vi "WriteConnInfoUSB.vi"(8 "error in (no error)":errorcluster, 9 "hostname":string="ConnectionInfo.json", 10 "path":path, 11 "connection info":T1) -> (0 "error out":errorcluster)   [LabVIEW 2017, in "USBDrive.lvlib"]
uses:
  <vilib>/addons/InsightCM/Devices/Shared/Common/USBDrive/USBDrive.lvlib
  <vilib>/addons/InsightCM/MessageBus/Base/controls/ConnectionInfo.ctl
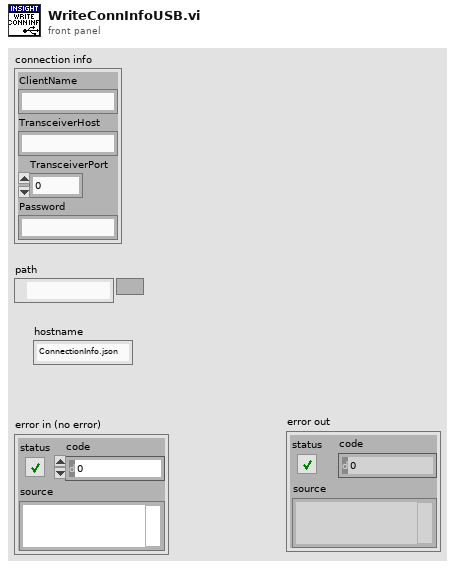
[diagram p1: front panel]
types:
  T1 = typedef "ConnectionInfo.ctl" = cluster{"ClientName":string, "TransceiverHost":string, "TransceiverPort":u16, "Password":string}
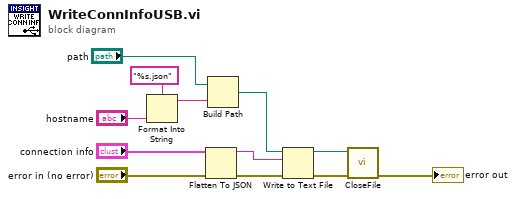
[diagram p0: block diagram]
diagram:
  n1 = Format Into String(format string="%s.json", "hostname") -> (resulting string=w8:string)  [unwired: 2 in, 1 out]
  n2 = Flatten To JSON(anything="connection info", error in (no error)="error in (no error)") -> (JSON string=w9:string, 11:w12:errorcluster)  [unwired: 1 in]
  n3 = Build Path(base path="path", name or relative path=w8) -> (appended path=w10:path)
  n4 = Write to Text File(file (use dialog)=w10, text=w9, error in=w12) -> (refnum out=w3:refnum<file>, error out=w2:errorcluster)  [unwired: 1 in, 1 out]
  n5 = call <vilib>:"CloseFile.vi"("error in (no error)"=w2, "file reference"=w3) -> ("error out"=→"error out":errorcluster)  [unwired: 9 in]
